vi "TestRobSteerAdjust.vi"() -> ()   [LabVIEW 2014]
panel:
  out "Set Out":dbl
  in  "Encoder":dbl
  in  "Axes":dbl[](array[numeric])
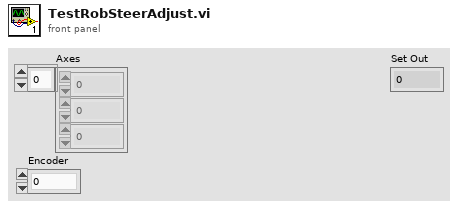
[diagram p1: front panel]
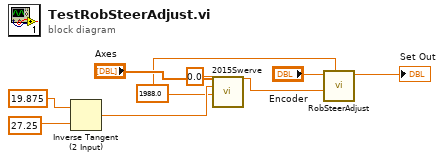
[diagram p0: block diagram]
diagram:
  w2 = 1988.0 ("EncoderTicksPerRev")
  n1 = Inverse Tangent (2 Input)(1:27.25 ("Robot Width"), 2:19.875 ("Robot Length")) -> (0:w6:dbl)
  n2 = call "2015Swerve.vi"("Axes"="Axes", "Robot Dimension Calc"=w6, "EncoderTicksPerRev"=w2, "Encoder Offset"=0.0) -> ("FL Angle"=w4:dbl)  [unwired: 16 in, 7 out]
  n3 = call "RobSteerAdjust.vi"("EncoderTicksPerRev"=w2, "Set In"=w4, "Encoder"="Encoder") -> ("Set Out"=→"Set Out":dbl)  [unwired: 8 in]
